vi "Beep (SubVI).vi"(11 "Numeric":dbl) -> ()   [LabVIEW 2021]
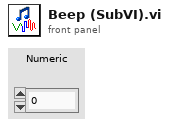
[diagram p1: front panel]
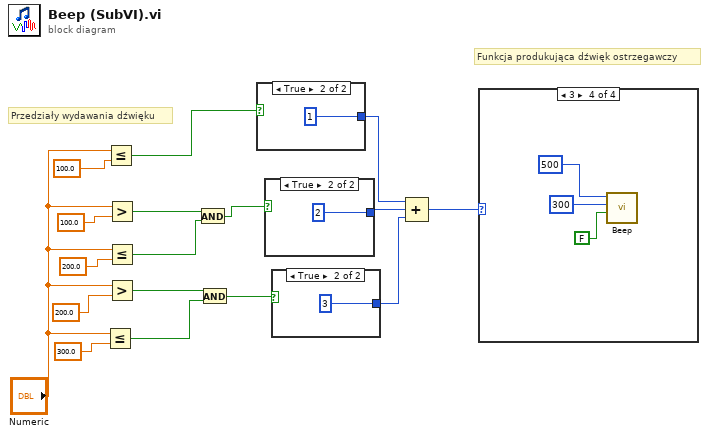
[diagram p0: block diagram]
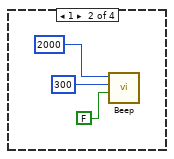
[diagram p3: hidden frame]
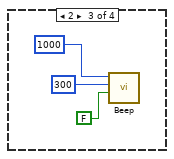
[diagram p4: hidden frame]
diagram:
  # "Funkcja produkująca dźwięk ostrzegawczy"
  # "Przedziały wydawania dźwięku"
  n1 = Less Or Equal?(x="Numeric", y=300.0) -> (x <= y?=w9:bool)
  n2 = Less Or Equal?(x="Numeric", y=100.0) -> (x <= y?=w10:bool)
  n3 = Greater?(x="Numeric", y=100.0) -> (0:w3:bool)
  n4 = Less Or Equal?(x="Numeric", y=200.0) -> (x <= y?=w5:bool)
  n5 = Greater?(x="Numeric", y=200.0) -> (0:w7:bool)
  n6 = And(x=w3, y=w5) -> (x .and. y?=w11:bool)
  n7 = And(x=w7, y=w9) -> (x .and. y?=w12:bool)
  n8 = case shown="True" w10 {
    tunnel: [_ 1] -> w13
    frame False {
    }
    frame True {
    }
  }
  n9 = case shown="True" w11 {
    tunnel: [_ 2] -> w15
    frame False {
    }
    frame True {
    }
  }
  n10 = case shown="True" w12 {
    tunnel: [_ 3] -> w14
    frame False {
    }
    frame True {
    }
  }
  n11 = Compound Arithmetic op=ADD(w13, w15, w14) -> (w16:i32)
  n12 = case shown="3" w16 {
    frame 0, Default {
    }
    frame 1 {
      n13 = call <vilib>:"Beep.vi"("use system alert? (T)"=FALSE, "duration (msec)"=u32 300, "frequency (Hz)"=u32 2000) -> ()  [unwired: 9 in]
    }
    frame 2 {
      n14 = call <vilib>:"Beep.vi"("use system alert? (T)"=FALSE, "duration (msec)"=u32 300, "frequency (Hz)"=u32 1000) -> ()  [unwired: 9 in]
    }
    frame 3 {
      n15 = call <vilib>:"Beep.vi"("use system alert? (T)"=FALSE, "duration (msec)"=u32 300, "frequency (Hz)"=u32 500) -> ()  [unwired: 9 in]
    }
  }
